vi "tsdiag_can_communication_control.vi"(7 "ATimeOutMs":i32, 8 "错误输入（无错误）":errorcluster, 9 "AControlType":u8, 10 "ADiagModuleIndex":i32, 11 "Path":path) -> (0 "错误输出":errorcluster, 2 "Return Type":i32, 3 "Path output":path)   [LabVIEW 2014]
doc: "Function Introduction :\nSet CAN communication control type\nCall location :\ninput parameter :\nADiagModulus Index: Handle to UDS module\nACControlType: Communication Control Type\nReturn value :\n==0: Execution successful\nOther values: Query error code"
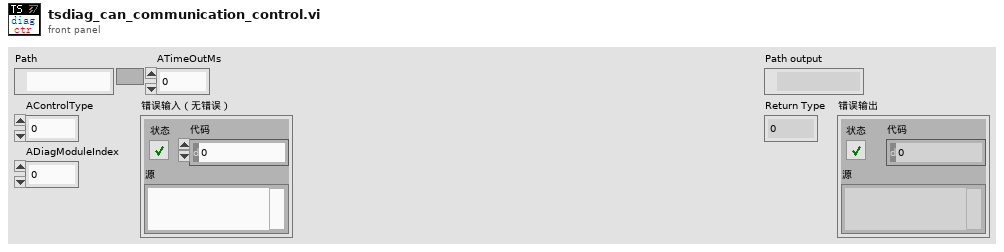
[diagram p1: front panel]
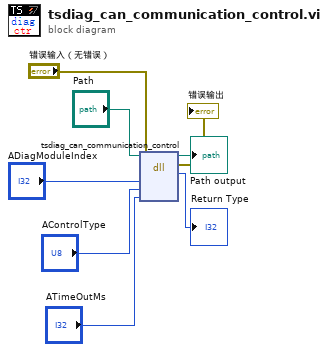
[diagram p0: block diagram]
diagram:
  n1 = dll-call lib="C:/Users/XYY/Desktop/LabView Demo/TSCAN_LB2018_V1.4_20220309/Config/TSMaster.dll" fn="tsdiag_can_communication_control"(path in="Path", error in="错误输入（无错误）", "ADiagModuleIndex"="ADiagModuleIndex", "AControlType"="AControlType", "ATimeOutMs"="ATimeOutMs") -> (path out=→"Path output":path, error out=→"错误输出":errorcluster, "返回类型"=→"Return Type":i32)  [unwired: 4 in]
